vi "Mecanum Drive.vi"(0 "X In":dbl, 5 "Y In":dbl, 7 "R In":dbl, 9 "Manual Override":bool, 11 "Reset Header":bool) -> (4 "X Out":dbl, 6 "Y Out":dbl, 8 "R Out":dbl)   [LabVIEW 2014]
uses:
  <vilib>/addons/control/pid/pid.llb/PID (DBL).vi
  <vilib>/addons/control/pid/NI_PID_pid.lvlib
panel:
  out "Header":dbl
  out "Initialize Header":bool=TRUE
  in  "STRAIGHT PID":T1={"proportional gain (Kc)"=0.02, "integral time (Ti, min)"=0.05, "derivative time (Td, min)"=0.0} {"derivative time (Td, min)" format="%.3f"; "integral time (Ti, min)" format="%.3f"; "proportional gain (Kc)" format="%.3f"}
  out "PID Output":dbl format="%.2f"
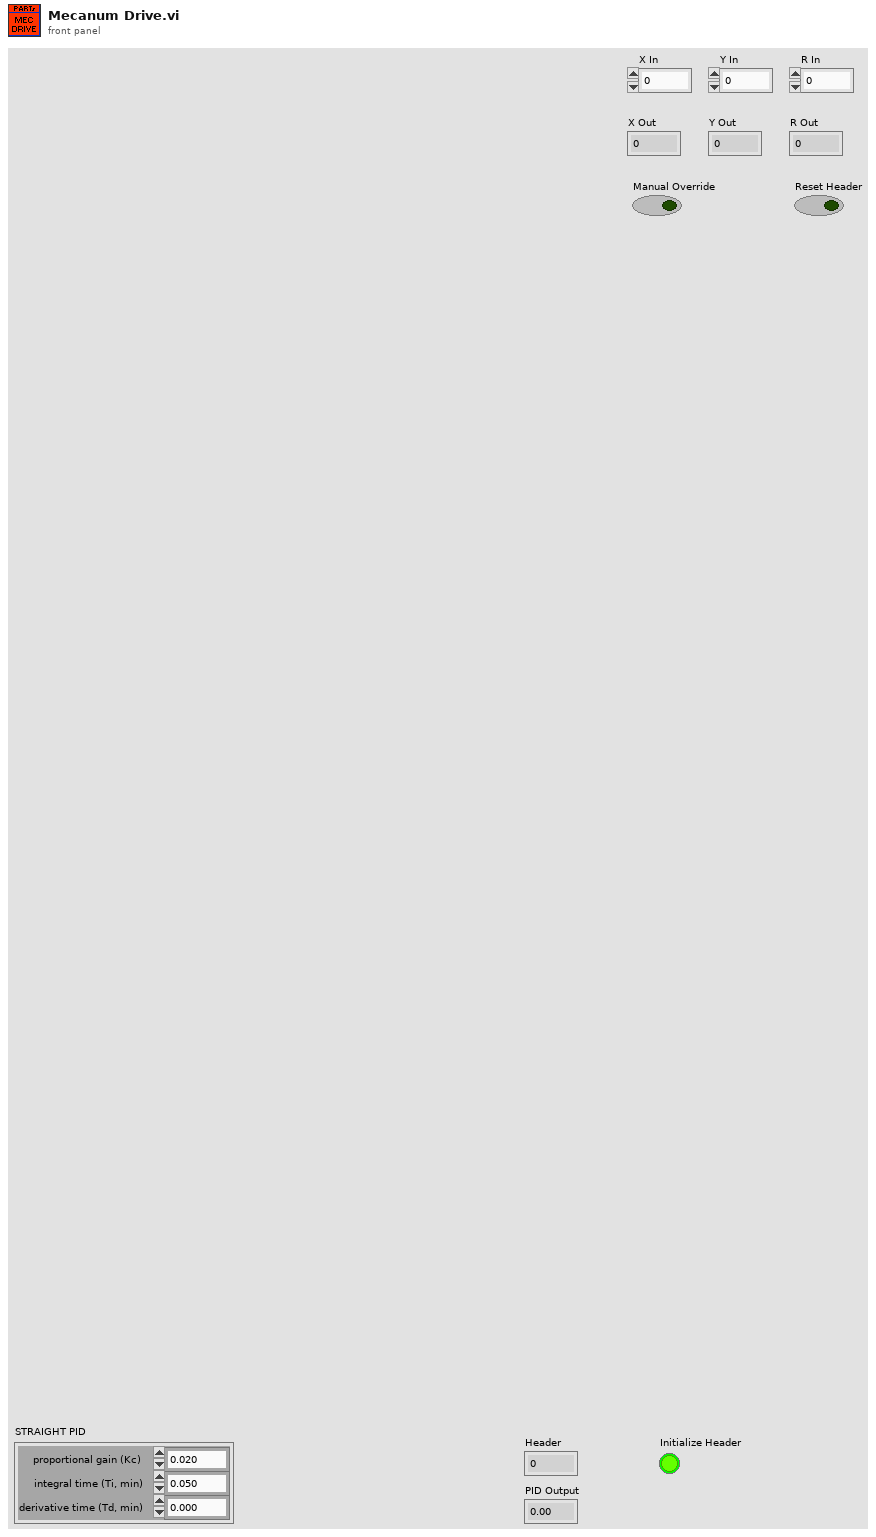
[diagram p1: front panel]
types:
  T1 = cluster{"proportional gain (Kc)":dbl, "integral time (Ti, min)":dbl, "derivative time (Td, min)":dbl}
  T2 = typedef "WPI_GyroDevRef.ctl" = cluster{"DevStatus":errorcluster, "Analog Module":T3, "Analog Channel":T4, "Offset":dbl, "Gain (VoltsPerDegree/Second)":dbl}
  T3 = typedef "FPGA_TypedefAnalogModule.ctl" = enum16{"Controller 1"}
  T4 = typedef "FPGA_AIChannel.ctl" = enum8{"AI 0", "AI 1", "AI 2", "AI 3", "AI MXP 0", "AI MXP 1", "AI MXP 2", "AI MXP 3", "Invalid"}
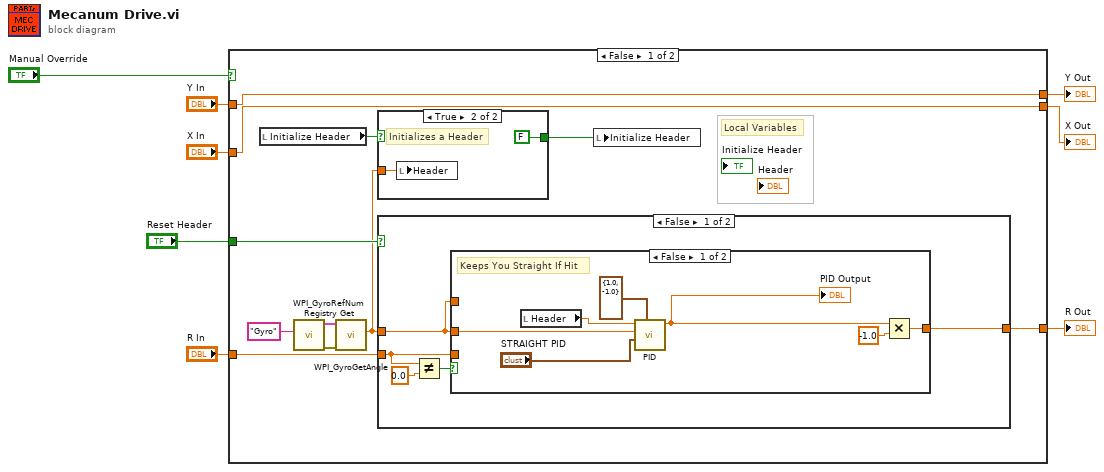
[diagram p0: block diagram]
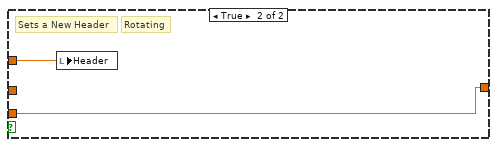
[diagram p2: hidden frame]
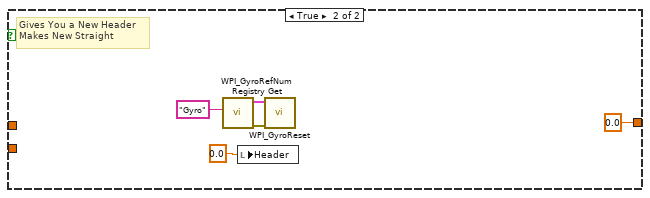
[diagram p3: hidden frame]
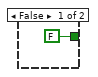
[diagram p4: hidden frame]
diagram:
  n1 = case shown="False" "Manual Override" {
    tunnel: [w19 w42] -> w2
    tunnel: "Y In" -> [w9 w44]
    tunnel: "X In" -> [w10 w43]
    tunnel: "Reset Header" -> [w16 _]
    tunnel: [w9 w44] -> w3
    tunnel: "R In" -> [w11 w42]
    tunnel: [w10 w43] -> w4
    frame False {
      # "Local Variables"
      n2 = local read "Initialize Header"() -> (w18:bool)
      n3 = call <vilib>:"WPI_GyroRefNum Registry Get.vi"("refnum name"="Gyro") -> ("error out"=w12:errorcluster, "GyroDevRef"=w14:T2)  [unwired: 9 in]
      n4 = call <vilib>:"WPI_GyroGetAngle.vi"("error in (no error)"=w12, "GyroDevRef"=w14) -> ("Angle"=w13:dbl)  [unwired: 6 in, 3 out]
      n5 = case shown="True" w18 {
        tunnel: w13 -> [_ w41]
        tunnel: [FALSE FALSE] -> w17
        frame False {
        }
        frame True {
          # "Initializes a Header"
          n6 = local write "Header"(w41) -> ()
        }
      }
      n7 = case shown="False" w16 {
        tunnel: [w24 0.0] -> w19
        tunnel: w11 -> [w21 _]
        tunnel: w13 -> [w20 _]
        frame False {
          n8 = Not Equal?(x=w21, y=0.0) -> (x != y?=w22:bool)
          n9 = case shown="False" w22 {
            tunnel: [w30 w32] -> w24
            tunnel: w20 -> [w31 _]
            tunnel: w20 -> [_ w33]
            tunnel: w21 -> [_ w32]
            frame False {
              # "Keeps You Straight If Hit"
              n10 = local read "Header"() -> (w27:dbl)
              n11 = call-poly <vilib>:"PID.vi"("output range"=cluster{"output high":dbl, "output low":dbl} {"output high"=1.0, "output low"=-1.0}, "PID gains"="STRAIGHT PID", "process variable"=w31, "setpoint"=w27) -> ("output"=w26:dbl)  [unwired: 6 in, 1 out]
              "PID Output" <- w26
              n12 = Multiply(x=w26, y=-1.0) -> (x*y=w30:dbl)
            }
            frame True {
              # "Sets a New Header"
              # "Rotating"
              n13 = local write "Header"(w33) -> ()
            }
          }
        }
        frame True {
          # "Gives You a New Header\nMakes New Straight"
          n14 = call <vilib>:"WPI_GyroRefNum Registry Get.vi"("refnum name"="Gyro") -> ("error out"=w37:errorcluster, "GyroDevRef"=w36:T2)  [unwired: 9 in]
          n15 = local write "Header"(0.0 ("Header 2")) -> ()
          n16 = call <vilib>:"WPI_GyroReset.vi"("error in (no error)"=w37, "GyroDevRef"=w36) -> ()  [unwired: 8 in, 2 out]
        }
      }
      n17 = local write "Initialize Header"(w17) -> ()
    }
    frame True {
    }
  }
  "X Out" <- w4
  "Y Out" <- w3
  "R Out" <- w2
